vi "新建.vi"(8 "error in (no error)":errorcluster caption="错误输入（无错误）", 11 "路径":path) -> (0 "error out":errorcluster caption="错误输出", 3 "数据文件.lvclass":refnum<class "数据文件.lvclass">)   [LabVIEW 2021, in "数据文件.lvclass"]
doc: "本VI是为《我和LabVIEW》一书编写的示例。\n关于本书的介绍请参考网页：\nhttp://ruanqizhen.spaces.live.com/blog/cns!5852D4F797C53FB6!4310.entry"
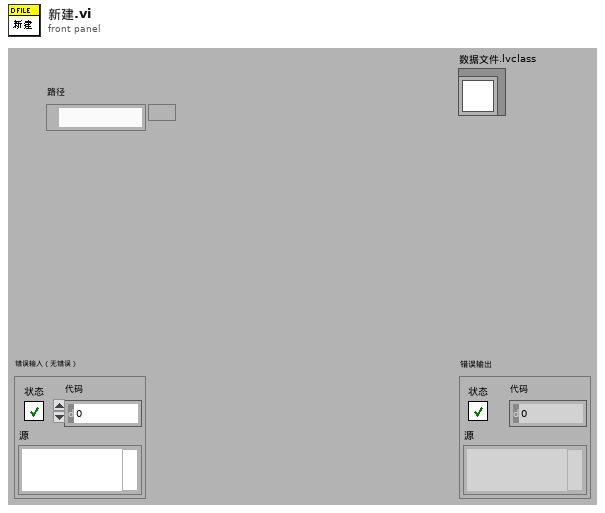
[diagram p1: front panel]
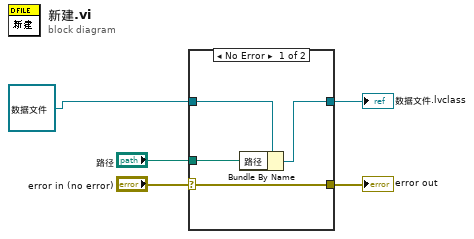
[diagram p0: block diagram]
diagram:
  n1 = case shown="No Error" "error in (no error)" {
    selector: "error in (no error)" -> [w8 w11]
    tunnel: [w8 w11] -> w4
    tunnel: [w7 w10] -> w3
    tunnel: refnum<class "数据文件.lvclass"> refnum ("数据文件.lvclass") -> [w9 w10]
    tunnel: "路径" -> [w6 _]
    frame No Error {
      n2 = Bundle By Name(cluster=w9, "路径"=w6) -> (w7:refnum<class "数据文件.lvclass">)
    }
    frame Error {
    }
  }
  "error out" <- w4
  "数据文件.lvclass" <- w3
